vi "DKc_2024.vi"(0 "Temperature / K":dbl=293.16 format="%.4g", 1 "Type of air":i32(listbox)=4, 2 "xw water mol. fract.":dbl=0.011584, 3 "CO2 content (ppm)":dbl=368.0) -> (4 "DCp0":dbl=4.243658129143587e-05 format="%.6f", 5 "DKc/1+Kc":dbl=4.8312433834734244e-06 format="%#.2g", 6 "DCp0/Cp0 rel. unc. CP0/R humid air":dbl=1.210528326419047e-05 format="%.6g", 7 "DKc":dbl=4.836261191873891e-06 format="%.7f", 8 "Kc - correzione":dbl=-0.0010386163565326845 format="%.6g")   [LabVIEW 2016]
panel:
  out "Cp0/R humid air":dbl=3.5056248057383876 format="%.6f"
  # "±"
  # "±"
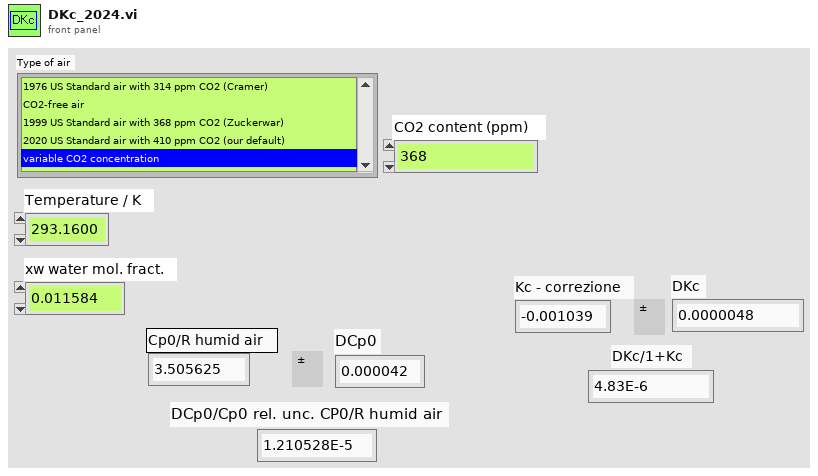
[diagram p1: front panel]
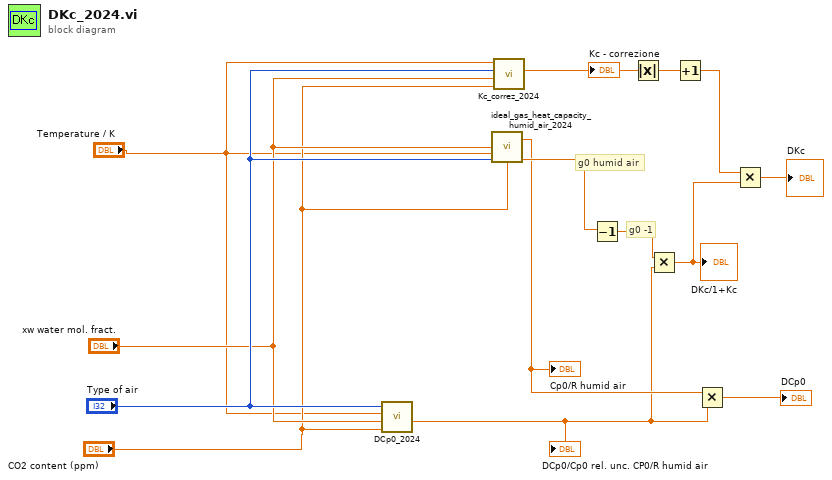
[diagram p0: block diagram]
diagram:
  # "g0 -1"
  # "g0 humid air"
  n1 = call "DCp0_2024.vi"("CO2 content (ppm)"="CO2 content (ppm)", "molar fraction of water vapor"="xw water mol. fract.", "Temperature / K"="Temperature / K", "Type of air"="Type of air") -> ("rel. unc. Cp0 humid air"=w2:dbl)  [unwired: 5 in, 2 out]
  "DCp0/Cp0 rel. unc. CP0/R humid air" <- w2
  n2 = call "ideal_gas_heat_capacity_humid_air_2024.vi"("molar fraction of water vapor"="xw water mol. fract.", "Temperature [K]"="Temperature / K", "Type of air"="Type of air", "CO2 content (ppm)"="CO2 content (ppm)") -> ("Cp0/R humid air"=w9:dbl, "Gamma0 humid air"=w14:dbl)  [unwired: 2 in, 8 out]
  "Cp0/R humid air" <- w9
  n3 = call "Kc_correz_2024.vi"("Temperature [K]"="Temperature / K", "Type of air"="Type of air", "H2O molar fraction"="xw water mol. fract.", "CO2 content (ppm)"="CO2 content (ppm)") -> ("Kc - correction"=w7:dbl)  [unwired: 5 out]
  "Kc - correzione" <- w7
  n4 = Decrement(x=w14) -> (x-1=w13:dbl)
  n5 = Absolute Value(x=w7) -> (abs(x)=w6:dbl)
  n6 = Multiply(x=w13, y=w2) -> (x*y=w12:dbl)
  "DKc/1+Kc" <- w12
  n7 = Increment(x=w6) -> (x+1=w11:dbl)
  n8 = Multiply(x=w9, y=w2) -> (x*y=→"DCp0":dbl)
  n9 = Multiply(x=w11, y=w12) -> (x*y=→"DKc":dbl)
